vi "Glyph to Bitmap Glyph.vi"(8 "error in (no error)":errorcluster, 10 "Offset":cluster{"x":sgl, "y":sgl}, 11 "glyph ref in":i64) -> (0 "error out":errorcluster, 2 "bitmap glyph ref out":i64, 3 "glyph ref out":i64)   [LabVIEW 2023, in "Freetype Drawer.lvlib"]
uses:
  Freetype Drawer.lvlib
  libfreetype.dll
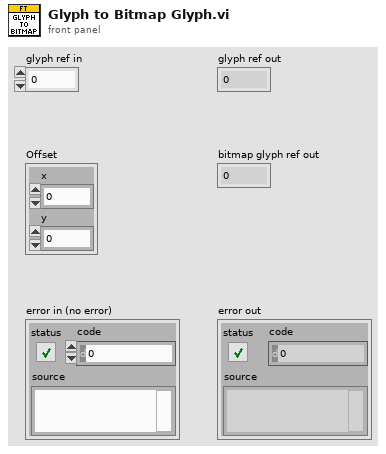
[diagram p1: front panel]
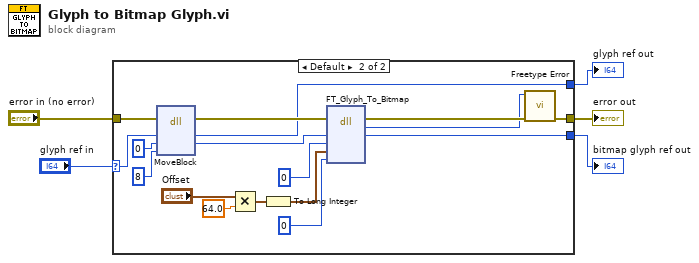
[diagram p0: block diagram]
diagram:
  n1 = case shown="Default" "glyph ref in" {
    selector: "glyph ref in" -> [w6 w24]
    tunnel: "error in (no error)" -> [w7 w17]
    tunnel: [w7 w16] -> w3
    tunnel: [_ w13] -> w2
    tunnel: [w6 w12] -> w1
    frame 0 {
    }
    frame Default {
      n2 = dll-call lib="LabVIEW" fn="MoveBlock"(error in=w17, "src"=w24, "dst"=i64 0 ("render_mode"), "size"=8) -> (error out=w20:errorcluster, "src"=w12:i64, "dst"=w23:i64)  [unwired: 4 in, 1 out]
      n3 = Multiply(x="Offset", y=sgl 64.0) -> (x*y=w11:cluster{"x":sgl, "y":sgl})
      n4 = To Long Integer(number=w11) -> (32bit integer=w9:cluster{"x":i32, "y":i32})
      n5 = dll-call lib="E:/Labview/LV 2023/Libs/LV Symbol/Freetype Drawer/libfreetype.dll" fn="FT_Glyph_To_Bitmap"(error in=w20, "glyph ref"=w23, "render_mode"=0, "origin"=w9, "destroy"=0) -> (error out=w18:errorcluster, "error"=w15:i32, "glyph ref"=w13:i64)  [unwired: 5 in, 1 out]
      n6 = call "Freetype Error.vi"("error in (no error)"=w18, "Error"=w15) -> ("error out"=w16:errorcluster)  [unwired: 9 in]
    }
  }
  "error out" <- w3
  "bitmap glyph ref out" <- w2
  "glyph ref out" <- w1
